vi "Config Serial Port.vi"(8 "error in (no error)":errorcluster, 10 "Timeout (3sec)":u32=3000, 11 "VISA resource name":refnum<visa-resource-name>) -> (0 "error out":errorcluster, 3 "VISA resource name out":refnum<visa-resource-name>)   [LabVIEW 2015, in "XYZStage.lvlib"]
uses:
  XYZStage.lvlib
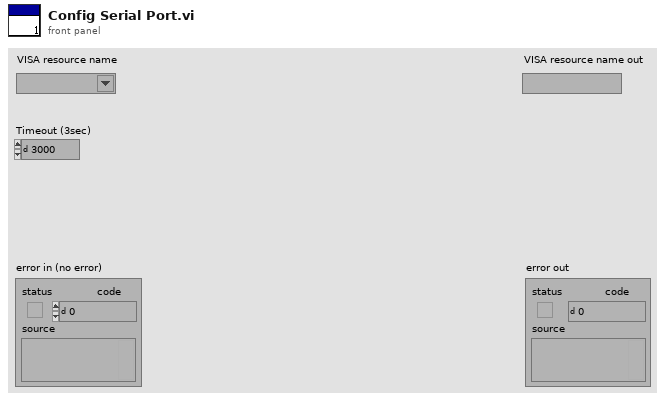
[diagram p1: front panel]
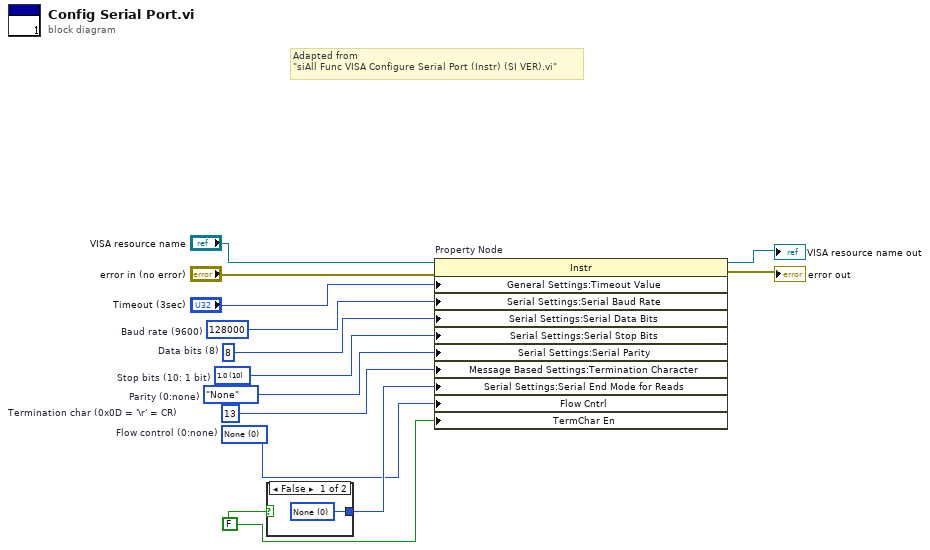
[diagram p0: block diagram]
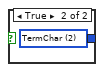
[diagram p2: hidden frame]
diagram:
  w1 = FALSE ("Enable Termination Char (F)")
  w2 = u16 0 items=["None", "XON/XOFF", "RTS/CTS", "XON/XOFF & RTS/CTS", "DTR/DSR", "XON/XOFF & DTR/DSR"]  # Flow control (0:none)
  w9 = u8 13  # Termination char (0x0D = '\r' = CR)
  w10 = enum16{"None", "Odd", "Even", "Mark", "Space"}."None"  # Parity (0:none)
  w4 = u16 10 items=["1.0"=10, "1.5"=15, "2.0"=20]  # Stop bits (10: 1 bit)
  w11 = u16 8  # Data bits (8)
  w12 = u32 128000  # Baud rate (9600)
  # "Adapted from\n\"siAll Func VISA Configure Serial Port (Instr) (SI VER).vi\""
  n1 = case shown="False" w1 {
    tunnel: [w14 w15] -> w3
    frame False {
      w14 = u16 0 items=["None", "LastBit", "TermChar"] ("Serial Settings:Serial End Mode for Reads")
    }
    frame True {
      w15 = u16 2 items=["None", "LastBit", "TermChar"] ("Serial Settings:Serial End Mode for Reads")
    }
  }
  n2 = property on="Property Node" class="Instr"(reference="VISA resource name", error in="error in (no error)", "General Settings:Timeout Value"="Timeout (3sec)", "Serial Settings:Serial Baud Rate"=w12, "Serial Settings:Serial Data Bits"=w11, "Serial Settings:Serial Stop Bits"=w4, "Serial Settings:Serial Parity"=w10, "Message Based Settings:Termination Character"=w9, "Serial Settings:Serial End Mode for Reads"=w3, "Flow Cntrl"=w2, "TermChar En"=w1) -> (reference out=→"VISA resource name out":refnum<visa-resource-name>, error out=→"error out":errorcluster)
